vi "Listbox.vi"() -> ()   [LabVIEW 2023]
doc: "Demonstrates the use of the Listbox control."
panel:
  out "Multiple Selections":string[](array[string])
  out "Multiple Selection Listbox Value":i32[](array[numeric])
  in  "Multiple Selection Listbox":i32[](listbox)=[0, 2, 4]
  out "Single Selection":string
  out "Single Selection Listbox Value":i32
  in  "Single Selection Listbox":i32(listbox)
  # "Overview: Demonstrates the use of the Listbox control.\nInstructions:\n1. Select an item in the Single Selection Listbox.\n2. Select multiple items in the Multiple Selection Listbox by Ctrl-clicking the items (or Cmd-clicking on Mac OS).\n3. Run the VI. The values and names of the selected items are displayed."
  # "To change the listbox selection mode, right-click on the listbox and change the Selection Mode."
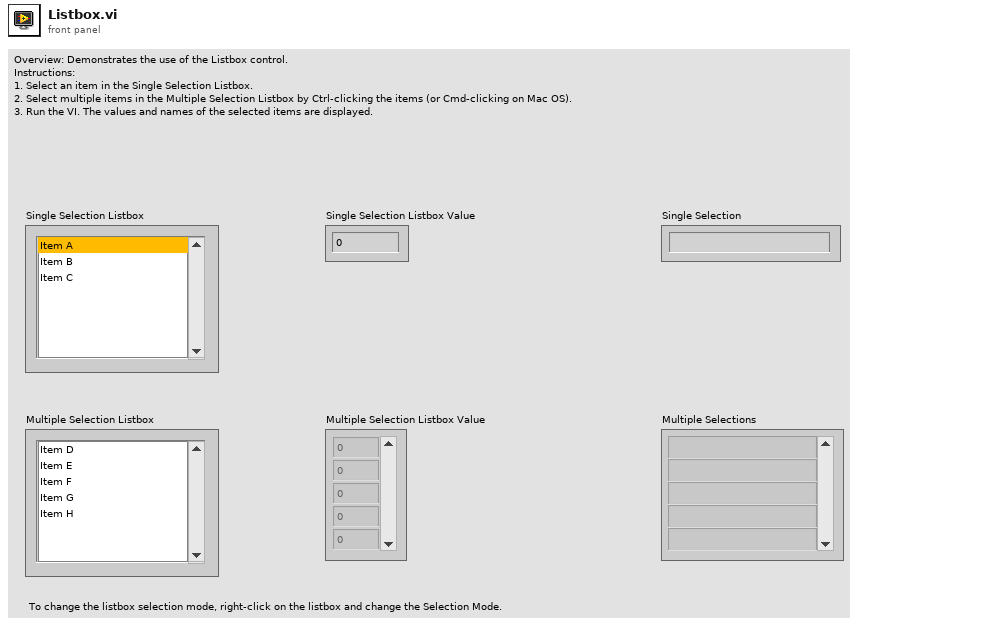
[diagram p1: front panel]
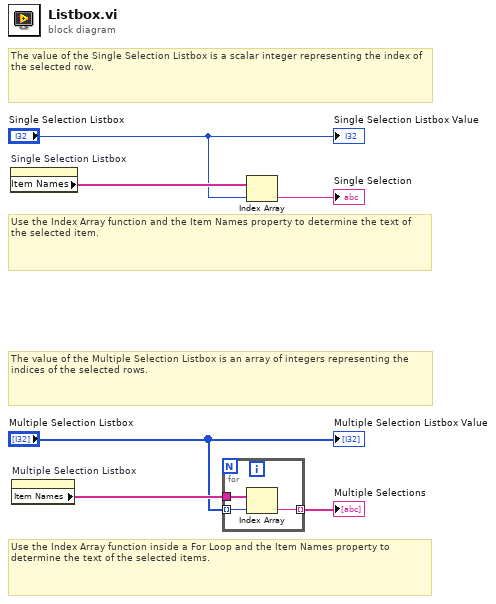
[diagram p0: block diagram]
diagram:
  # "Use the Index Array function inside a For Loop and the Item Names property to determine the text of the selected items."
  # "The value of the Multiple Selection Listbox is an array of integers representing the indices of the selected rows."
  # "Use the Index Array function and the Item Names property to determine the text of the selected item."
  # "The value of the Single Selection Listbox is a scalar integer representing the index of the selected row."
  n1 = property on="Single Selection Listbox" class="ListBox (strict)"() -> ("Item Names"=w6:string[])  [unwired: 2 in, 2 out]
  n2 = property on="Multiple Selection Listbox" class="LstBox (strict)"() -> ("Item Names"=w3:string[])  [unwired: 2 in, 2 out]
  n3 = for {
    tunnel: w3 -> [w9]
    tunnel: "Multiple Selection Listbox" -> [w8] mode=indexing
    tunnel: [w7] -> w1 mode=indexing
    n4 = Index Array(array=w9, index=w8) -> (element=w7:string)
  }
  "Multiple Selections" <- w1
  n5 = Index Array(array=w6, index="Single Selection Listbox") -> (element=→"Single Selection":string)
  "Single Selection Listbox Value" <- "Single Selection Listbox"
  "Multiple Selection Listbox Value" <- "Multiple Selection Listbox"
